vi "Fetch Multi Eval Meas SEM Margin Results.vi"(7 "Offset Frequency (Negative)":T1 items=["Negative", "Positive"], 8 "error in (no error)":errorcluster, 9 "Result Type (Current)":i32(ring) items=["Current"=0, "Average"=1, "Minimum"=5], 10 "Instance (1)":T2=1, 11 "VISA resource name":refnum<visa-resource-name>) -> (0 "error out":errorcluster, 1 "SEM Margin Results":cluster{"Margin X":dbl, "Margin Y":dbl}[](array[cluster]), 2 "Reliability":i32, 3 "VISA resource name out":refnum<visa-resource-name>, 4 "Out Of Tolerance":dbl format="%^.3e")   [LabVIEW 2020, in "Rohde&Schwarz CMXP NR FR2 Measurement.lvlib"]
doc: "Returns spectrum emission mask margin results. For each trace, the X and Y values of the margins for emission mask areas 1 to 12 are provided for negative and positive offset frequencies.\n\nAttributes:\nRSCMXPNRFR2M_ATTR_FETCH_MULTI_EVAL_MEASUREMENT_SEM_NEGATIVE_MARGIN_AVERAGE_RESULTS\nRSCMXPNRFR2M_ATTR_FETCH_MULTI_EVAL_MEASUREMENT_SEM_POSITIVE_MARGIN_AVERAGE_RESULTS\nRSCMXPNRFR2M_ATTR_FETCH_MULTI_EVAL_MEASUREMENT_SEM_NEGATIVE_MARGIN_CURRENT_RESULTS\nRSCMXPNRFR2M_ATTR_FETCH_MULTI_EVAL_MEASUREMENT_SEM_POSITIVE_MARGIN_CURRENT_RESULTS\nRSCMXPNRFR2M_ATTR_FETCH_MULTI_EVAL_MEASUREMENT_SEM_NEGATIVE_MARGIN_MINIMUM_RESULTS\nRSCMXPNRFR2M_ATTR_FETCH_MULTI_EVAL_MEASUREMENT_SEM_POSITIVE_MARGIN_MINIMUM_RESULTS\n\nRemote-control commands:\nFETCh:NRMMw:MEAS<i>:MEValuation:SEMask:MARGin:AVERage:NEGativ?\nFETCh:NRMMw:MEAS<i>:MEValuation:SEMask:MARGin:AVERage:POSitiv?\nFETCh:NRMMw:MEAS<i>:MEValuation:SEMask:MARGin:CURRent:NEGativ?\nFETCh:NRMMw:MEAS<i>:MEValuation:SEMask:MARGin:CURRent:POSitiv?\nFETCh:NRMMw:MEAS<i>:MEValuation:SEMask:MARGin:MINimum:NEGativ?\nFETCh:NRMMw:MEAS<i>:MEValuation:SEMask:MARGin:MINimum:POSitiv?"
uses:
  <instrlib>/Rohde&Schwarz CMXP NR FR2 Measurement/Rohde&Schwarz CMXP NR FR2 Measurement.lvlib
  <instrlib>/Rohde&Schwarz CMXP NR FR2 Measurement/Private/_Instance.ctl
  <instrlib>/Rohde&Schwarz CMXP NR FR2 Measurement/Private/_Offset Frequency.ctl
  <instrlib>/Rohde&Schwarz CMXP NR FR2 Measurement/Private/rsidr_core.llb/rsidr_core.lvlib
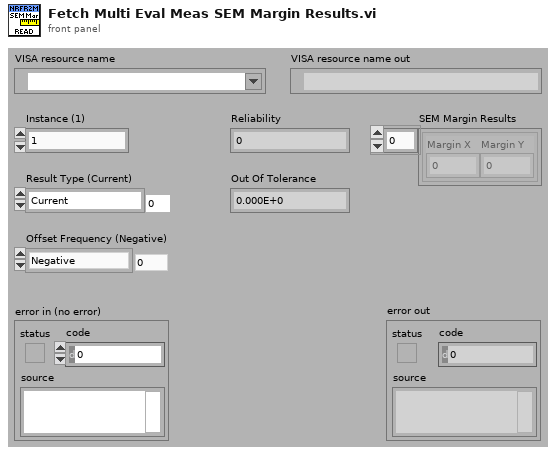
[diagram p1: front panel]
types:
  T1 = typedef "Rohde&Schwarz CMXP NR FR2 Measurement.lvlib/_Offset Frequency.ctl" = i32
  T2 = typedef "Rohde&Schwarz CMXP NR FR2 Measurement.lvlib/_Instance.ctl" = i32
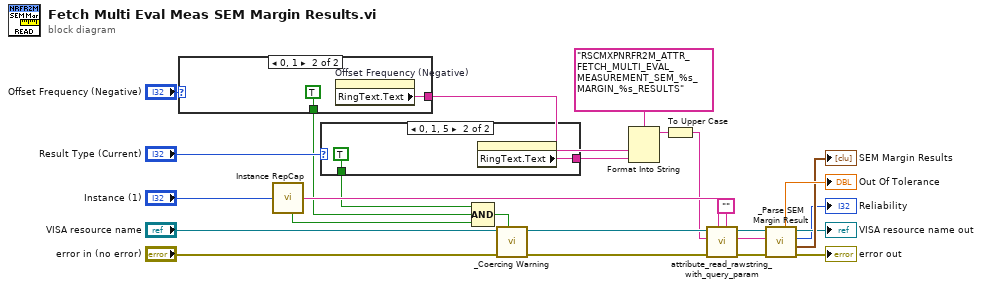
[diagram p0: block diagram]
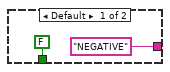
[diagram p2: hidden frame]
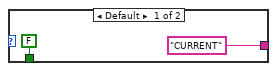
[diagram p3: hidden frame]
diagram:
  n1 = case shown="0, 1" "Offset Frequency (Negative)" {
    tunnel: ["NEGATIVE" w29] -> w4
    tunnel: [FALSE TRUE] -> w3
    frame Default {
    }
    frame 0, 1 {
      n2 = property on="Offset Frequency (Negative)" class="Ring (strict)"() -> ("RingText.Text"=w29:string)  [unwired: 2 in, 2 out]
    }
  }
  n3 = call <instrlib>:"Instance RepCap.vi"("Instance In"="Instance (1)") -> ("In Range?"=w8:bool, "RepCap Identifier Out"=w16:string)  [unwired: 1 in]
  n4 = case shown="0, 1, 5" "Result Type (Current)" {
    tunnel: ["CURRENT" w33] -> w9
    tunnel: [FALSE TRUE] -> w2
    frame Default {
    }
    frame 0, 1, 5 {
      n5 = property on="Result Type (Current)" class="Ring (strict)"() -> ("RingText.Text"=w33:string)  [unwired: 2 in, 2 out]
    }
  }
  n6 = Compound Arithmetic op=AND(w2, w3, w8) -> (w7:bool)
  n7 = call <instrlib>:"_Coercing Warning.vi"("In Range?"=w7, "error in (no error)"="error in (no error)", "VISA resource name"="VISA resource name") -> ("error out"=w18:errorcluster, "VISA resource name out"=w17:refnum<visa-resource-name>)  [unwired: 7 in]
  n8 = Format Into String(format string="RSCMXPNRFR2M_ATTR_FETCH_MULTI_EVAL_MEASUREMENT_SEM_%s_MARGIN_%s_RESULTS", w4, w9) -> (resulting string=w15:string)  [unwired: 2 in, 1 out]
  n9 = To Upper Case(1:w15) -> (0:w14:string)
  n10 = call <instrlib>:"attribute_read_rawstring_with_query_param.vi"("Query Parameter (None)"="" ("Empty String Constant"), "Repeated Capability"=w16, "error in"=w18, "Attribute ID"=w14, "VISA resource name"=w17) -> ("error out"=w11:errorcluster, "Raw String out"=w13:string, "VISA resource name out"=w12:refnum<visa-resource-name>)  [unwired: 4 in]
  n11 = call <instrlib>:"_Parse SEM Margin Result.vi"("error in (no error)"=w11, "Input String"=w13, "VISA resource name"=w12) -> ("error out"=→"error out":errorcluster, "Results"=→"SEM Margin Results":cluster{"Margin X":dbl, "Margin Y":dbl}[], "Reliability"=→"Reliability":i32, "VISA resource name out"=→"VISA resource name out":refnum<visa-resource-name>, "Out Of Tolerance"=→"Out Of Tolerance":dbl)  [unwired: 4 in]
